vi "CreateUINetworkStreamWriter.vi"(8 "ErrorIn":errorcluster, 11 "IP Address":string) -> (0 "ErrorOut":errorcluster, 3 "NtwrkStrmUIWrtrRefOut":refnum<k21>)   [LabVIEW 2018]
uses:
  RT/RT_MainQueueElements.ctl
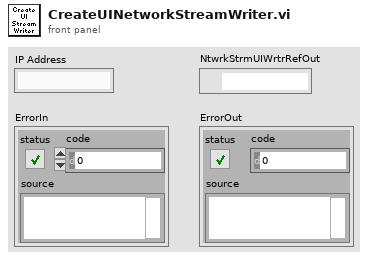
[diagram p1: front panel]
types:
  T1 = typedef "RT_MainQueueElements.ctl" = enum16{"Init", "Run", "ApplyTrggrs", "AbrtTrggrs", "ArmTrggrs", "ManTrggr", "Exit"}
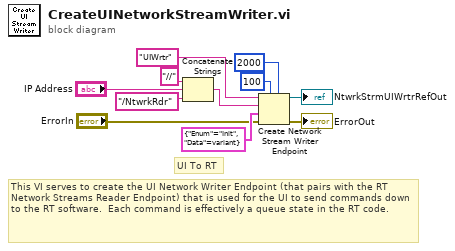
[diagram p0: block diagram]
diagram:
  # "This VI serves to create the UI Network Writer Endpoint (that pairs with the RT Network Streams Reader Endpoint) that is used for the UI to send commands down to the RT software.  Each command is effectively a queue state in the RT code."
  # "UI To RT"
  n1 = Concatenate Strings("//" ("string"), "IP Address", "/NtwrkRdr" ("string")) -> (w6:string)
  n2 = Create Network Stream Writer Endpoint(5:2000 ("writer buffer size"), 7:100 ("writer buffer size"), 8:"ErrorIn", 9:cluster{"Enum":T1, "Data":variant} {"Enum"=enum."Init", "Data"=variant} ("element"), 10:w6, 11:"UIWrtr" ("writer name")) -> (0:→"ErrorOut":errorcluster, 3:→"NtwrkStrmUIWrtrRefOut":refnum<k21>)  [unwired: 1 in]
